vi "Get Data.vi"(8 "error in (no error)":errorcluster, 11 "Serial IO in":refnum<class "Serial IO.lvclass">) -> (0 "error out":errorcluster, 2 "DataArray":refnum<class "Data.lvclass">[](array[class]), 3 "Serial IO out":refnum<class "Serial IO.lvclass">)   [LabVIEW 2015, in "Serial IO.lvclass"]
doc: "Retrieve data from the serial device. The data retrieved should be the standard data for the device, but the structure of that data may differ. This is the reason that an array of data class objects is returned rather than a single value."
uses:
  Serial IO.lvclass
  Data/Data.lvclass
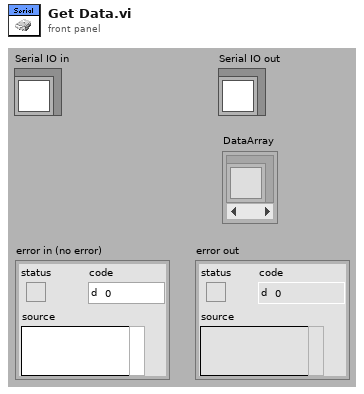
[diagram p1: front panel]
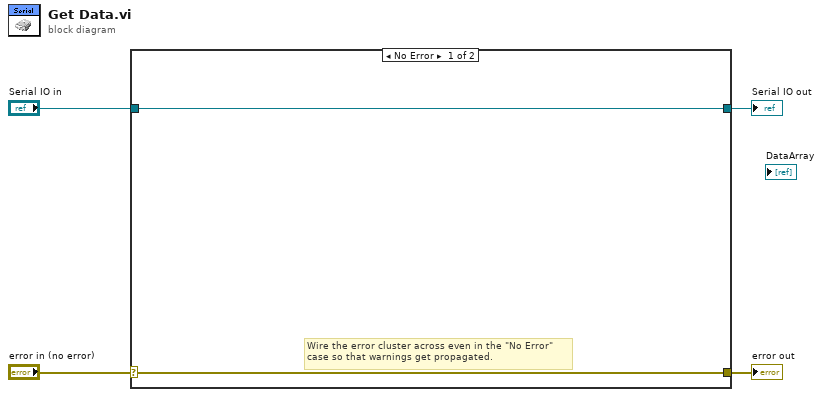
[diagram p0: block diagram]
diagram:
  n1 = case shown="No Error" "error in (no error)" {
    selector: "error in (no error)" -> [w5 w8]
    tunnel: [w5 w8] -> w3
    tunnel: [w6 w7] -> w1
    tunnel: "Serial IO in" -> [w6 w7]
    frame No Error {
      # "Wire the error cluster across even in the \"No Error\"\ncase so that warnings get propagated."
    }
    frame Error {
    }
  }
  "error out" <- w3
  "Serial IO out" <- w1
